vi "Open.vi"   [LabVIEW 2026, in "synnax_clib.lvlib" / "Synnax Writer.lvclass"]
uses:
  Synnax Writer.lvclass
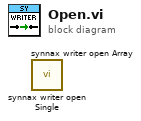
[diagram p0: block diagram]
diagram:
  n1 = call "synnax writer open Single.vi"() -> ()  [unwired: 9 in, 3 out]
  n2 = call "synnax writer open Array.vi"() -> ()  [unwired: 9 in, 3 out]
